vi "shuffle_2D.vi"(1 "Array IN":variant[][](array[variant])) -> (0 "Array OUT":variant[][](array[variant]))   [LabVIEW 2017, in "tools.lvlib"]
uses:
  tools.lvlib
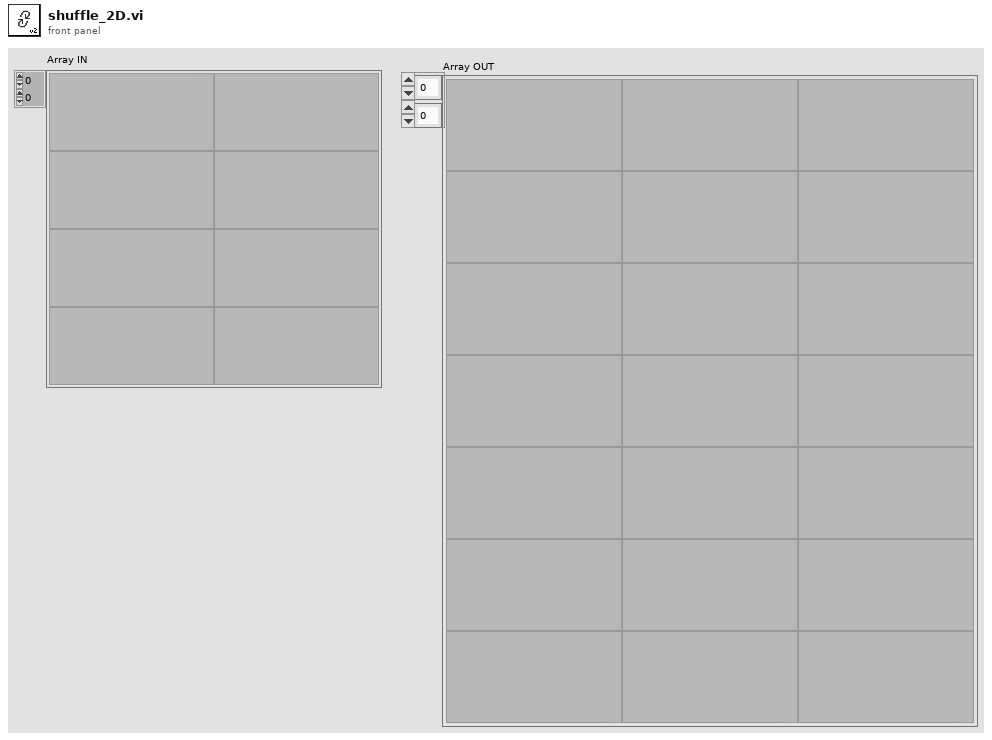
[diagram p1: front panel]
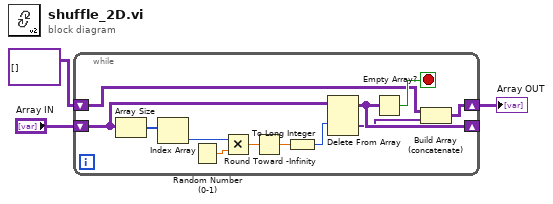
[diagram p0: block diagram]
diagram:
  n1 = while {
    shift-right: [w5] -> _
    shift-left: "Array IN" -> [w14]
    shift-right: [w11] -> w2
    shift-left: variant[][] [] -> [w12]
    stop <- w15 stop-if-true
    n2 = Array Size(array=w14) -> (size(s)=w7:i32[])
    n3 = Index Array(array=w7) -> (element=w6:i32)  [unwired: 1 in]
    n4 = Random Number (0-1)() -> (number: 0 to 1=w13:dbl)
    n5 = Multiply(x=w6, y=w13) -> (x*y=w10:dbl)
    n6 = Round Toward -Infinity(1:w10) -> (0:w9:dbl)
    n7 = To Long Integer(number=w9) -> (32bit integer=w8:i32)
    n8 = Delete From Array(array=w14, index (row)=w8) -> (deleted portion=w4:variant[], array with subset deleted=w5:variant[][])  [unwired: 2 in]
    n9 = Empty Array?(array=w5) -> (empty?=w15:bool)
    n10 = Build Array (concatenate)(w12, w4) -> (w11:variant[][])
  }
  "Array OUT" <- w2
